vi "datamsg(Reset).vi"   [LabVIEW 2014]
uses:
  <vilib>/FTP/NI_FTP.lvlib
types:
  T1 = typedef "NI_FTP.lvlib/FTP Session.ctl" = refnum<k5>
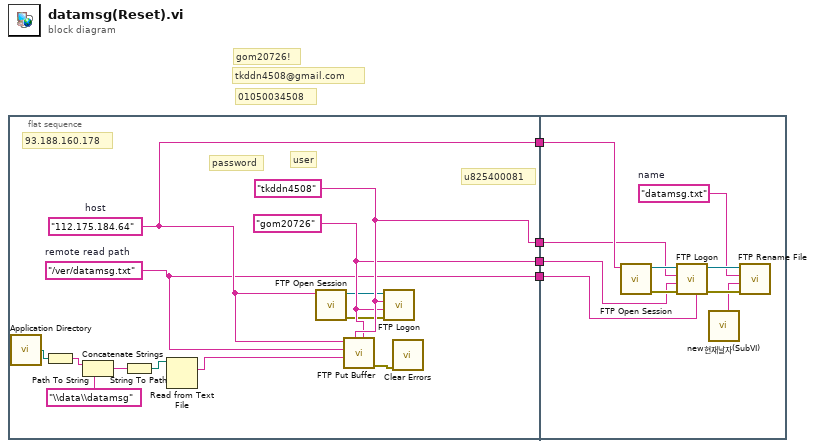
[diagram p0: block diagram]
diagram:
  # "gom20726!"
  # "01050034508"
  # "tkddn4508@gmail.com"
  n1 = flat-sequence {
    tunnel: [w16] -> w4
    tunnel: [w17] -> w3
    tunnel: [w15] -> w2
    tunnel: [w14] -> w1
    tunnel: w4 -> [w22]
    tunnel: w3 -> [w27]
    tunnel: w2 -> [w21]
    tunnel: w1 -> [w18]
    frame #0 {
      w15 = "gom20726"
      w16 = "tkddn4508"
      w14 = "/ver/datamsg.txt"  # remote read path
      w17 = "112.175.184.64"  # host
      # "u825400081"
      # "93.188.160.178"
      # "user"
      # "password"
      n2 = call <vilib>:"Application Directory.vi"() -> ("Application Directory"=w9:path)
      n3 = Path To String(path=w9) -> (string=w11:string)
      n4 = Concatenate Strings(w11, "\\data\\datamsg" ("문자열")) -> (w12:string)
      n5 = String To Path(string=w12) -> (path=w13:path)
      n6 = Read from Text File(file (use dialog)=w13) -> (text=w7:string)  [unwired: 3 in, 3 out]
      n7 = call <vilib>:"FTP Open Session.vi"("address"=w17) -> ("error out"=w5:errorcluster, "ftp session"=w6:T1)  [unwired: 7 in, 2 out]
      n8 = call <vilib>:"FTP Put Buffer.vi"("password"=w15, "user"=w16, "data"=w7, "remote path"=w14, "host"=w17) -> ("error out"=w8:errorcluster)  [unwired: 5 in, 1 out]
      n9 = call <vilib>:"FTP Logon.vi"("error in (no error)"=w5, "password"=w15, "user"=w16, "ftp session"=w6) -> ()  [unwired: 4 in, 4 out]
      n10 = call <vilib>:"Clear Errors.vi"("error in (no error)"=w8) -> ()  [unwired: 5 in, 2 out]
    }
    frame #1 {
      w20 = "datamsg.txt"  # name
      n11 = call <vilib>:"FTP Open Session.vi"("address"=w27) -> ("error out"=w25:errorcluster, "ftp session"=w26:T1)  [unwired: 7 in, 2 out]
      n12 = call <vilib>:"FTP Logon.vi"("starting path"=w18, "error in (no error)"=w25, "password"=w21, "user"=w22, "ftp session"=w26) -> ("error out"=w24:errorcluster, "ftp session out"=w23:T1)  [unwired: 3 in, 2 out]
      n13 = call "new현재날자(SubVI).vi"() -> ("날짜/시간 문자열"=w19:string)  [unwired: 5 in, 6 out]
      n14 = call <vilib>:"FTP Rename File.vi"("error in (no error)"=w24, "new name"=w19, "old name"=w20, "ftp session"=w23) -> ()  [unwired: 4 in, 4 out]
    }
  }
